vi "Update Hazards.vi"(9 "Map Input":dbl[][](array[numeric]), 10 "Hazard location":dbl[](array[numeric])) -> (3 "Map Output":dbl[][](array[numeric]))   [LabVIEW 2015]
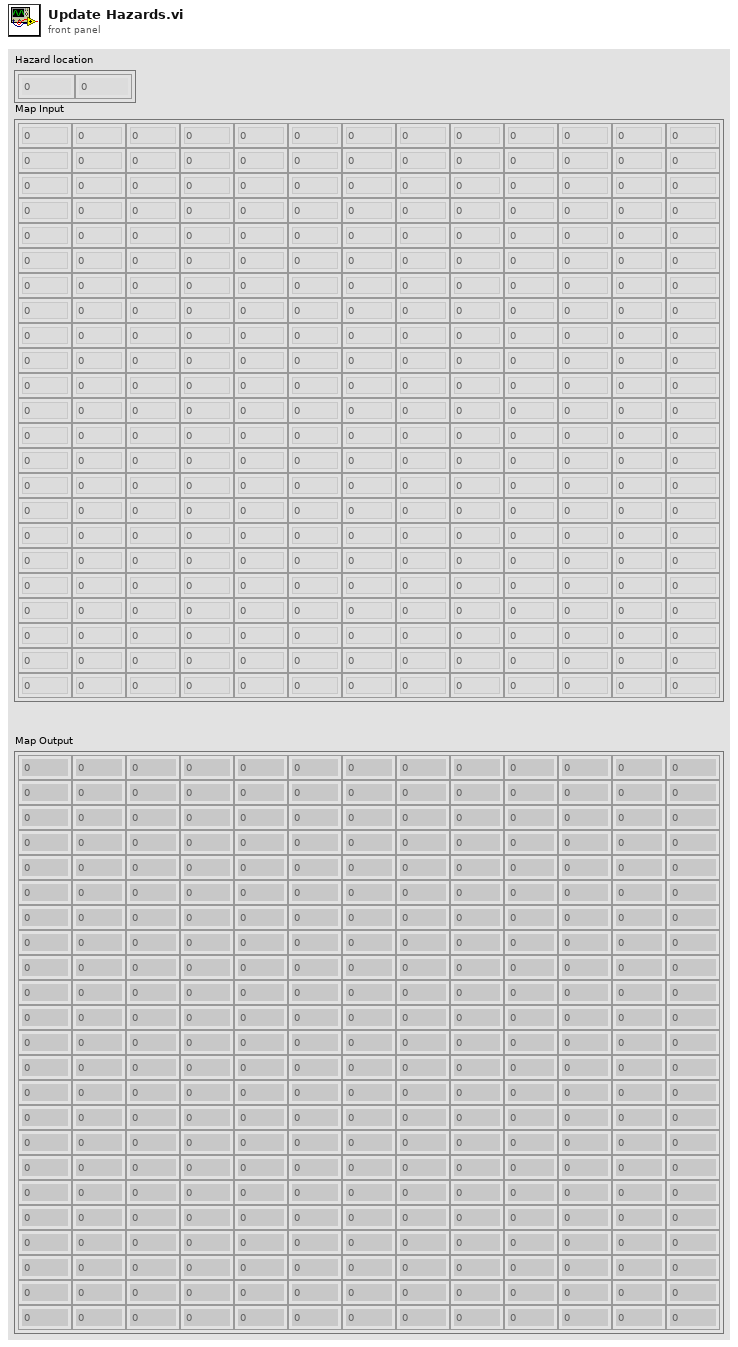
[diagram p1: front panel]
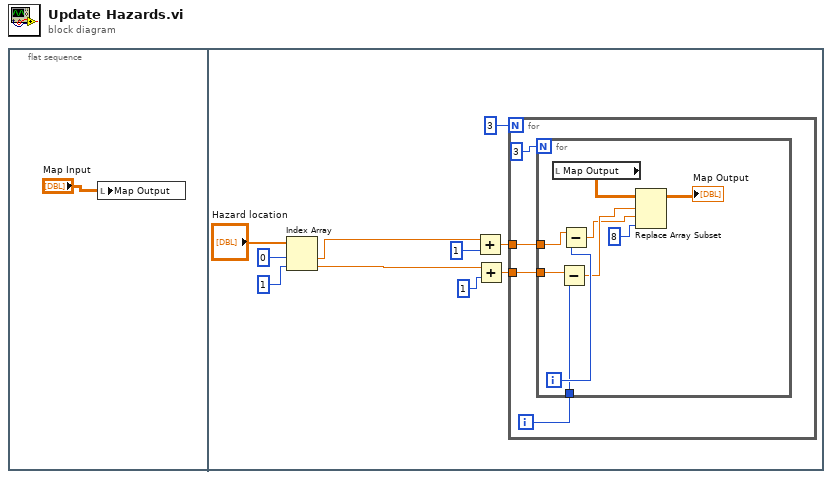
[diagram p0: block diagram]
diagram:
  n1 = flat-sequence {
    frame #0 {
      n2 = local write "Map Output"("Map Input") -> ()
    }
    frame #1 {
      n3 = Index Array(array="Hazard location", index #1=0, index #2=1) -> (element #1=w9:dbl, element #2=w10:dbl)
      n4 = Add(x=w9, y=1) -> (x+y=w7:dbl)
      n5 = Add(x=w10, y=1) -> (x+y=w8:dbl)
      n6 = for {
        N: 3 -> [_]
        tunnel: w7 -> [w14]
        tunnel: w8 -> [w13]
        i -> [w12]
        n7 = for {
          N: 3 -> [_]
          tunnel: w14 -> [w22]
          tunnel: w13 -> [w21]
          tunnel: w12 -> [w19]
          i -> [w20]
          n8 = local read "Map Output"() -> (w16:dbl[][])
          n9 = Subtract(x=w21, y=w19) -> (x-y=w18:dbl)
          n10 = Subtract(x=w22, y=w20) -> (x-y=w17:dbl)
          n11 = Replace Array Subset(array=w16, new element=8, index (row)=w18, index (col)=w17) -> (→"Map Output":dbl[][])
        }
      }
    }
  }
